vi "load protected file.vi"(8 "error in":errorcluster, 10 "password":string, 11 "Path":path) -> (0 "error out":errorcluster, 3 "data":string)   [LabVIEW 2016, in "lvlibretls configurable context.lvclass"]
uses:
  lvlibretls configurable context.lvclass
  lv tls dll.lvlib
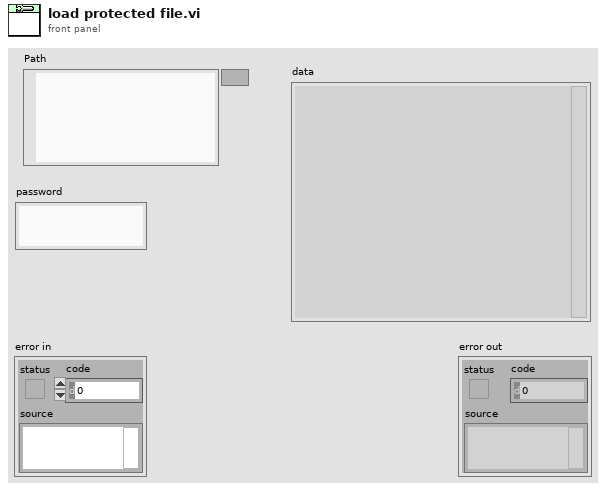
[diagram p1: front panel]
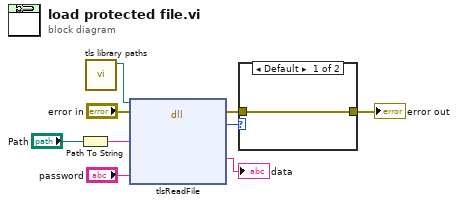
[diagram p0: block diagram]
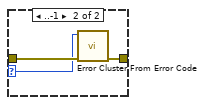
[diagram p2: hidden frame]
diagram:
  n1 = Path To String(path="Path") -> (string=w2:string)
  n2 = call "tls library paths.vi"() -> ("lvtls"=w1:path)  [unwired: 10 in, 1 out]
  n3 = dll-call lib="C:/Users/IEUser/Desktop/tlssimple/lvlibtls.dll" fn="tlsReadFile"(path in=w1, error in="error in", "filename"=w2, "password"="password") -> (error out=w8:errorcluster, "return"=w6:i32, "data"=→"data":string)  [unwired: 4 in, 1 out]
  n4 = case shown="Default" w6 {
    selector: w6 -> [_ w11]
    tunnel: w8 -> [w10 w13]
    tunnel: [w10 w12] -> w7
    frame Default {
    }
    frame ..-1 {
      n5 = call <vilib>:"Error Cluster From Error Code.vi"("error in (no error)"=w13, "error code (0)"=w11) -> ("error out"=w12:errorcluster)  [unwired: 7 in]
    }
  }
  "error out" <- w7
